vi "Acknowledge Fault.vi"(8 "Error In":errorcluster, 10 "Acknowledge Fault":bool, 11 "KIT-QVA in":refnum<class "KIT-QVA.lvclass">) -> (0 "Error Out":errorcluster, 3 "KIT-QVA out":refnum<class "KIT-QVA.lvclass">)   [LabVIEW 2014, in "KIT-QVA.lvlib" / "KIT-QVA.lvclass"]
doc: "Acknowledge fault."
uses:
  KIT-QVA.lvclass
  KIT-QVA.lvclass/KIT-QVA.ctl
  instr.lib/KIT-QV/KIT QV.lvlib
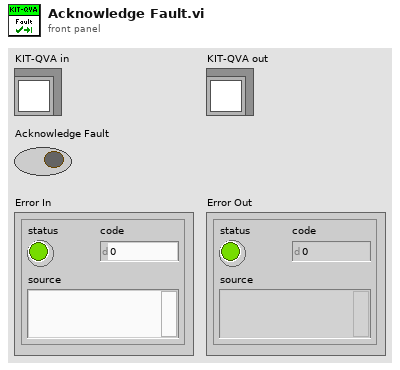
[diagram p1: front panel]
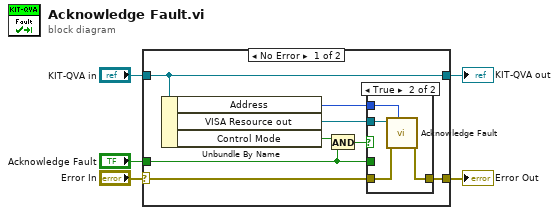
[diagram p0: block diagram]
diagram:
  n1 = case shown="No Error" "Error In" {
    selector: "Error In" -> [w10 w20]
    tunnel: [w9 w20] -> w4
    tunnel: [w13 w19] -> w2
    tunnel: "KIT-QVA in" -> [w13 w19]
    tunnel: "Acknowledge Fault" -> [w6 _]
    frame No Error {
      n2 = Unbundle By Name(w13) -> ("Address"=w11:u16, "VISA Resource out"=w12:refnum<visa-resource-name>, "Control Mode"=w8:bool)
      n3 = And(x=w8, y=w6) -> (x .and. y?=w7:bool)
      n4 = case shown="True" w7 {
        tunnel: w12 -> [_ w18]
        tunnel: w11 -> [_ w17]
        tunnel: w10 -> [w14 w16]
        tunnel: w6 -> [_ _]
        tunnel: [w14 w15] -> w9
        frame False {
        }
        frame True {
          n5 = call "Acknowledge Fault.vi"("Address"=w17, "Error In"=w16, "VISA Resource in"=w18) -> ("Error Out"=w15:errorcluster)  [unwired: 7 in, 1 out]
        }
      }
    }
    frame Error {
    }
  }
  "Error Out" <- w4
  "KIT-QVA out" <- w2
